vi "CheckForError.Test.vi"(0 "Main Path":path) -> (1 "Array of Folders":path[](array[path]), 2 "PRAMMS VRN":refnum<visa-resource-name>, 3 "Array of Files":path[](array[path]), 4 "SkipInstr":bool, 6 "Bundle-Meteo":T1={"cRIO address"="0.0.0.0", "Port Number"=0, "cRIO_commID"=refnum, "Cx"=FALSE}, 8 "This VI's Path":path, 10 "term":string, 11 "Go on ?":bool, 12 "Array of Baud Rates":u32[](array[numeric]), 13 "TCS-CommVRN":refnum<visa-resource-name>, 14 "Array of VISA refnum":refnum<visa-resource-name>[](array[refnum]), 15 "Serial":bool[](array[boolean]))   [LabVIEW 2011]
uses:
  Globals.vi
  <vilib>/Utility/config.llb/Read Key (U32).vi
  <vilib>/Utility/config.llb/Read Key (String).vi
  <vilib>/Instr/_visa.llb/VISA Configure Serial Port (Instr).vi
  Comm/SerialCommError.vi
  <vilib>/Utility/config.llb/Read Key (Path).vi
  <vilib>/Utility/config.llb/NI_LVConfig.lvlib
panel:
  in  "SkipInstr":bool
  out "Hexapode":bool
  out "Hexapod VRN":refnum<visa-resource-name>
  out "PRAMMS":bool
  out "ActiveDummy":bool
  out "TCS":bool
  out "TCP Error":errorcluster
  out "standard output":string
  out "standard error":string
  out "concatenated string":string
  out "Nettoyage":bool
  in  "restart":bool
  out "error out":errorcluster
  in  "cancel":bool
  in  "ignore":bool
  out "Master Dir":path
  out "IDL":bool
  out "wget":bool
  out "Ports Series":bool
  out "SubVIs":bool
  out "config error out":errorcluster
  out "Camera":bool
  out "Starry Night":bool
  out "Configuration":bool
  out "Arborescence":bool
  # "Version sans GUI de ErrorCheck.vi  Vérifie :\n    - Existence des chemins/fichiers nécessaire\n    - Communication avec les différents périphériques\n    - Lien ActiveX avec Starry Night\n    - Vérifie la communication avec la station météo\n    - Vérifie l'état de la face avant des VIs utilisés\n    - Compatibilité des versions installées\n    - Vérifie la disponibilité des applications (wget, IDL)"
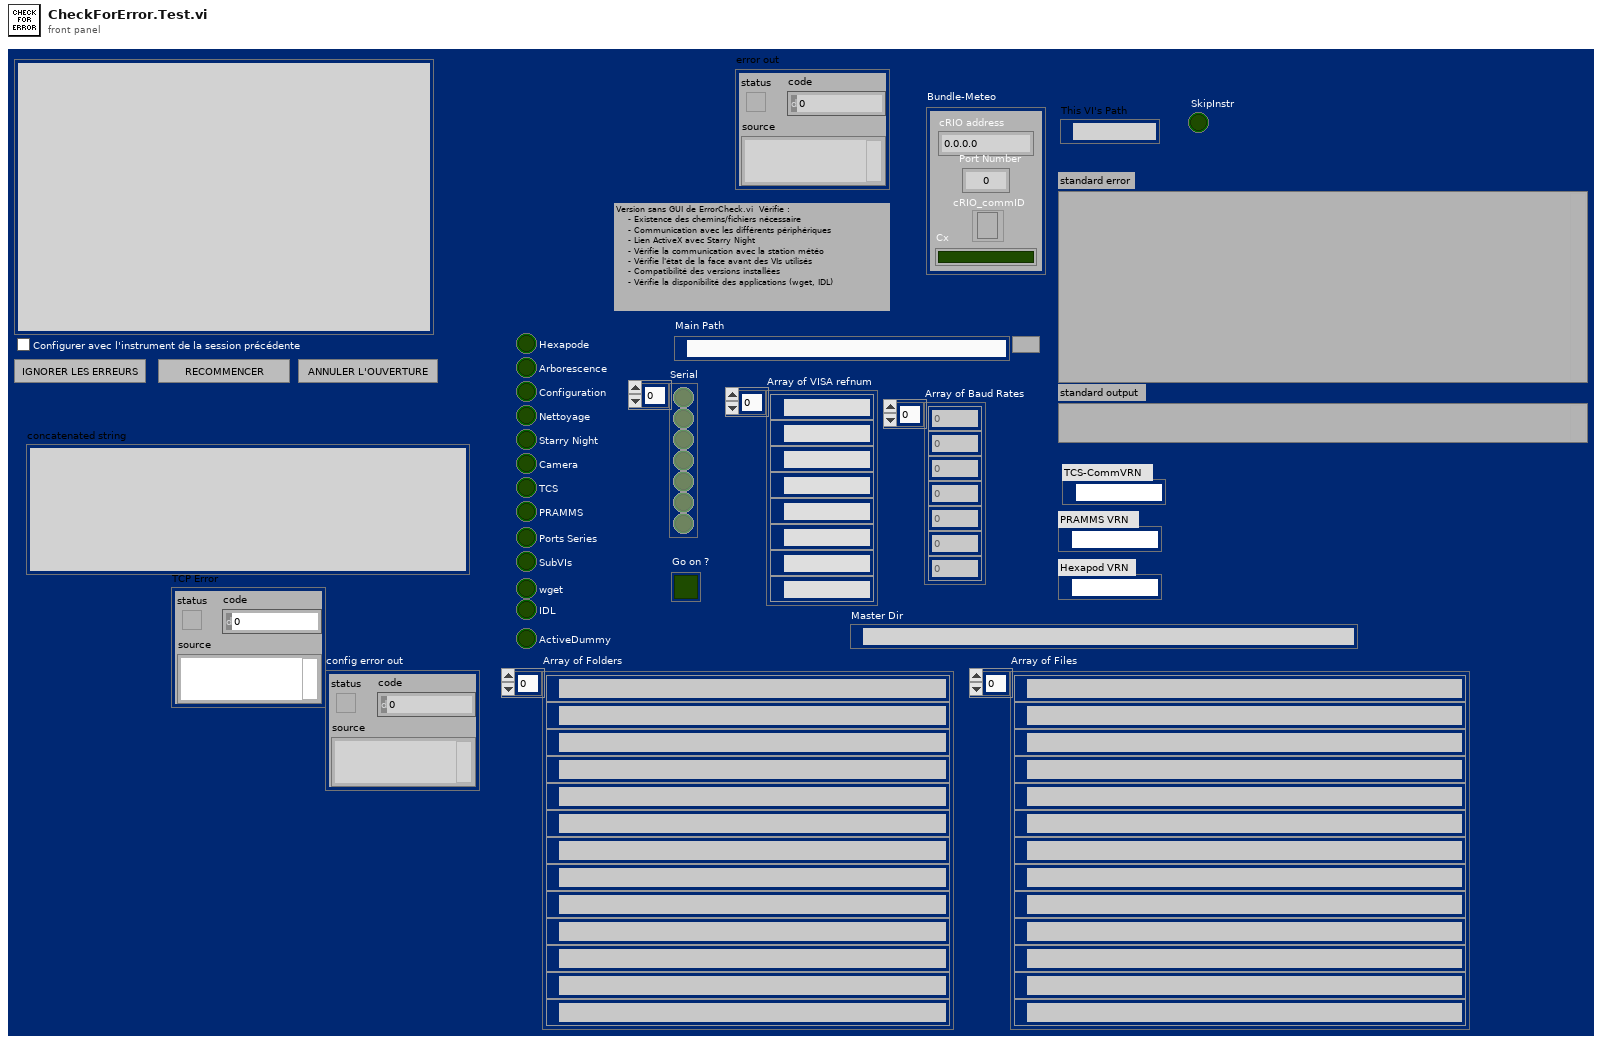
[diagram p1: front panel]
types:
  T1 = cluster{"cRIO address":string, "Port Number":u16, "cRIO_commID":refnum<k5>, "Cx":bool}
  T2 = enum8{"Enabled", "Disabled", "Disabled and Grayed Out"}
  T3 = typedef "NI_LVConfig.lvlib/Config Data RefNum.ctl" = refnum<k1>
  T4 = cluster{"value":string, u16, "connection ID":refnum<k5>, bool}
  T5 = enum16{"Left Button", "Center Button", "Right Button", "Window Close"}
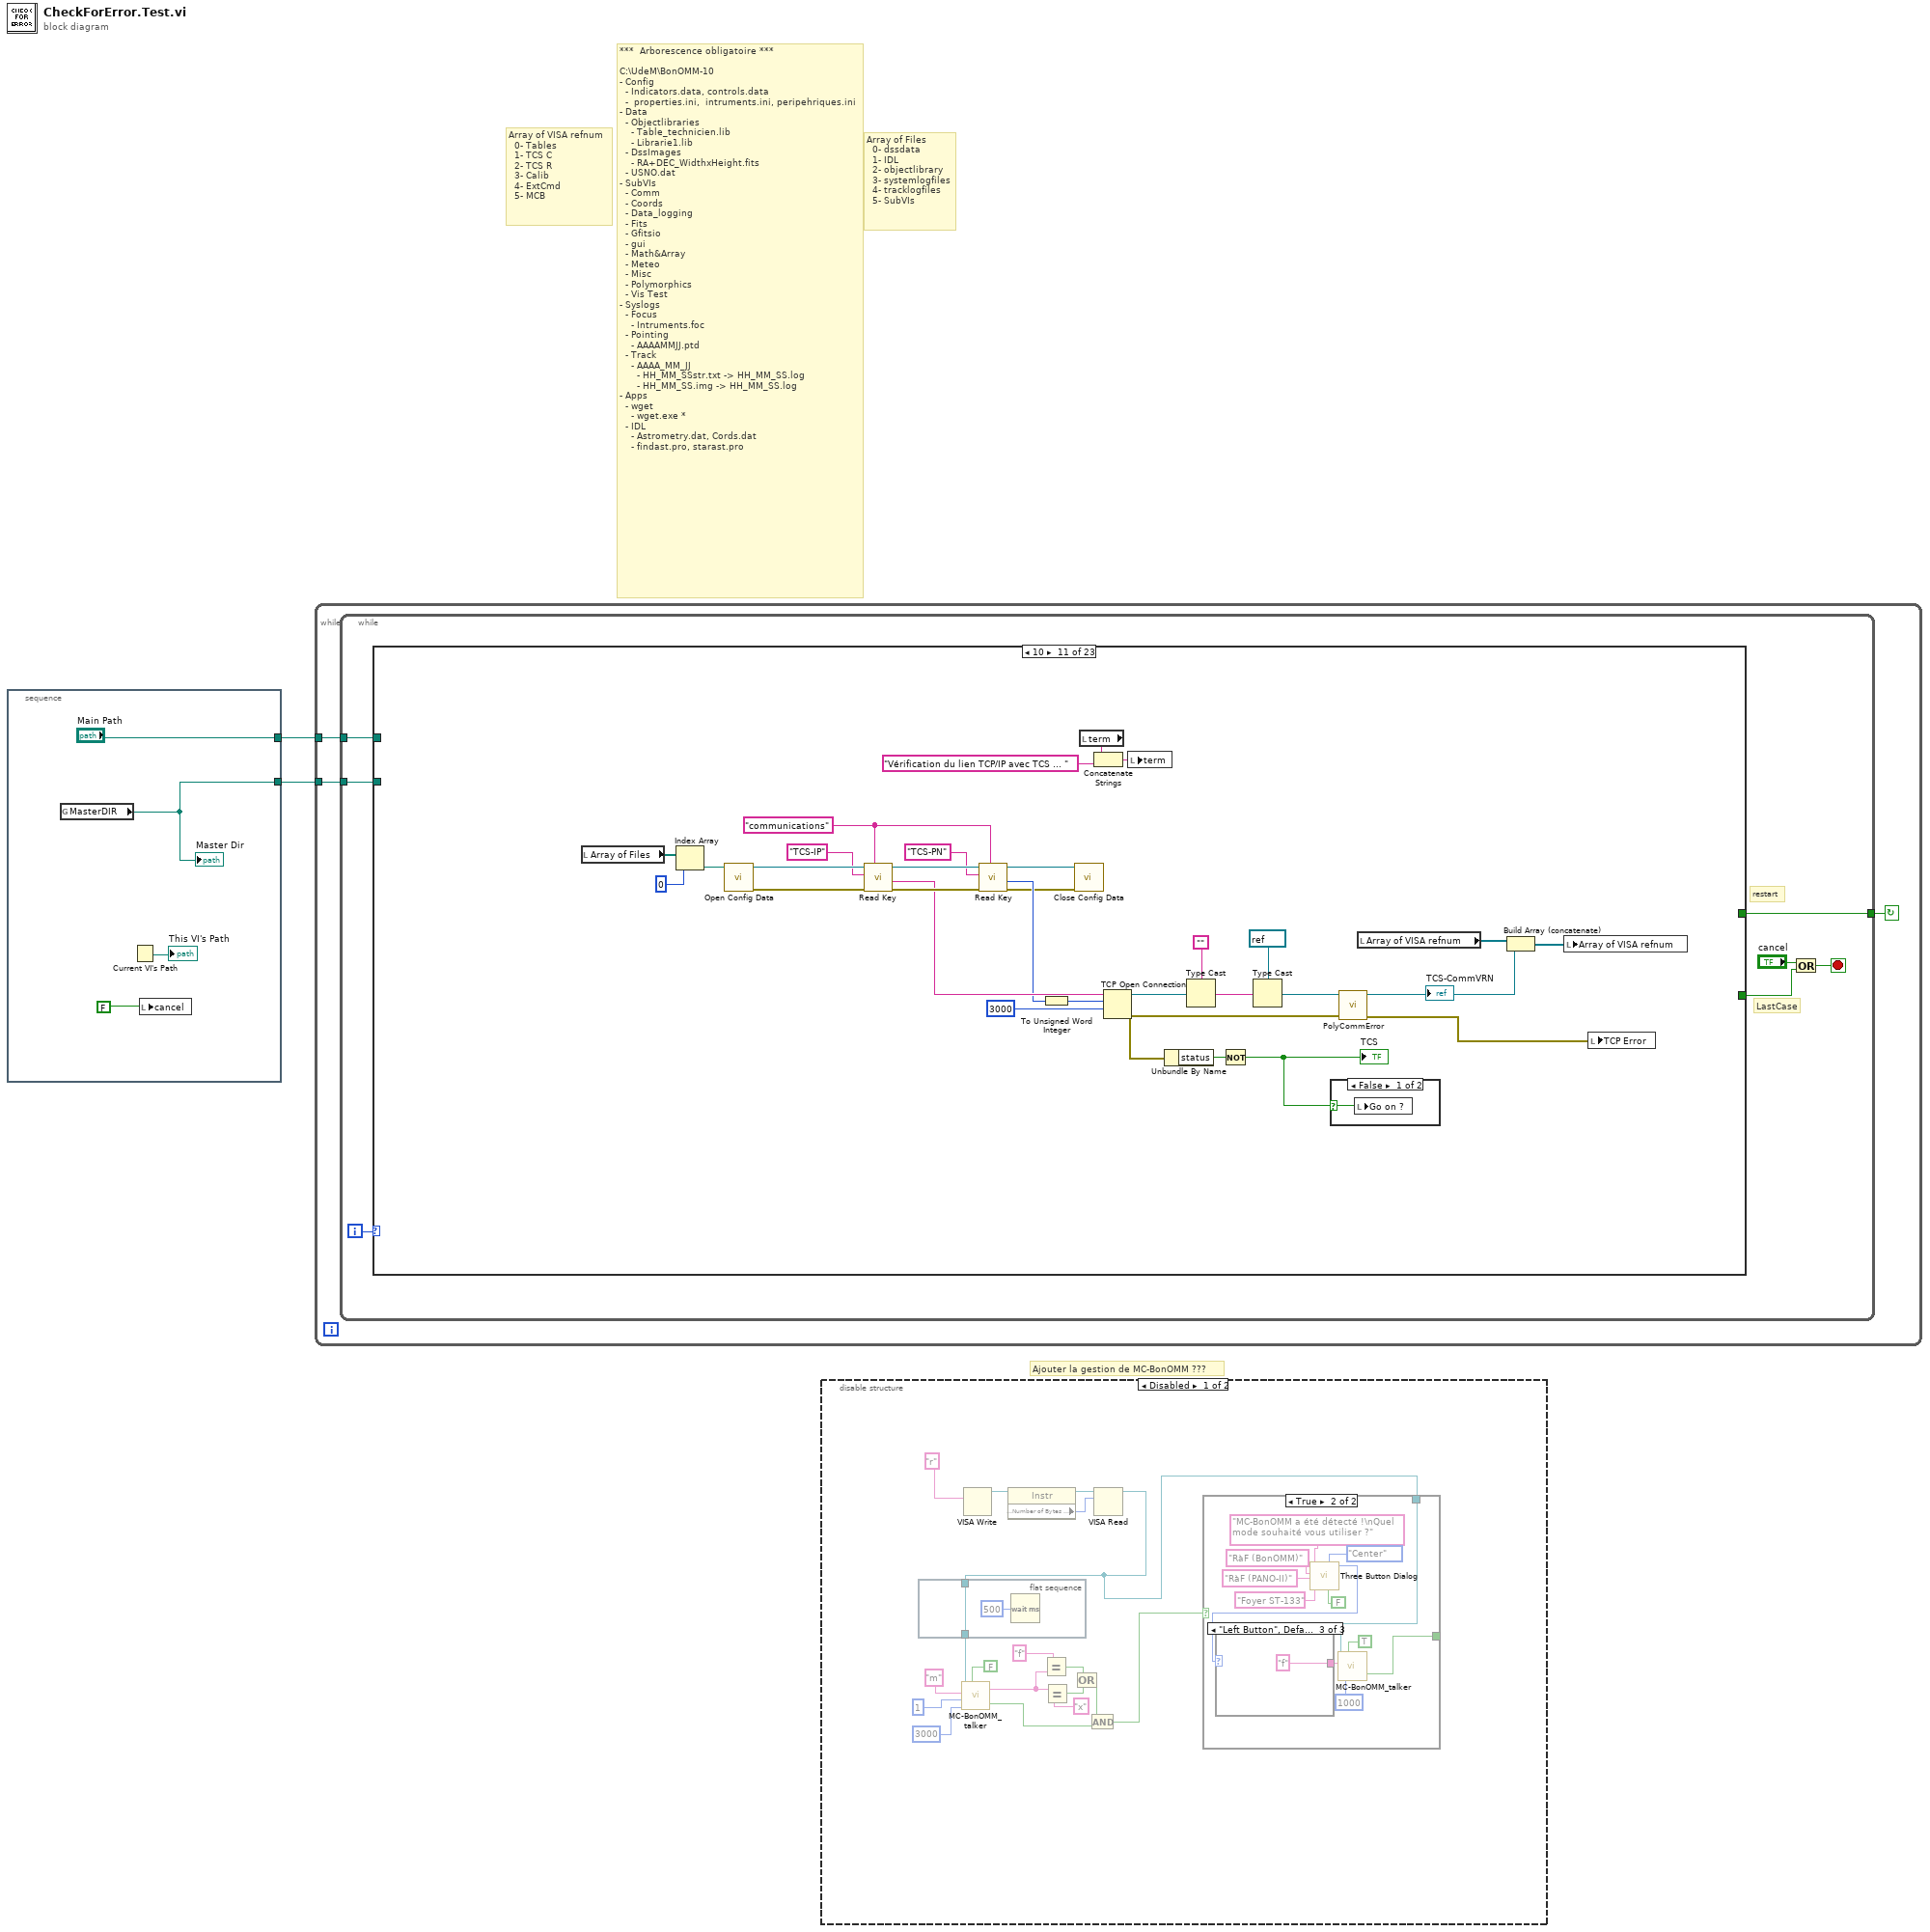
[diagram p0: block diagram]
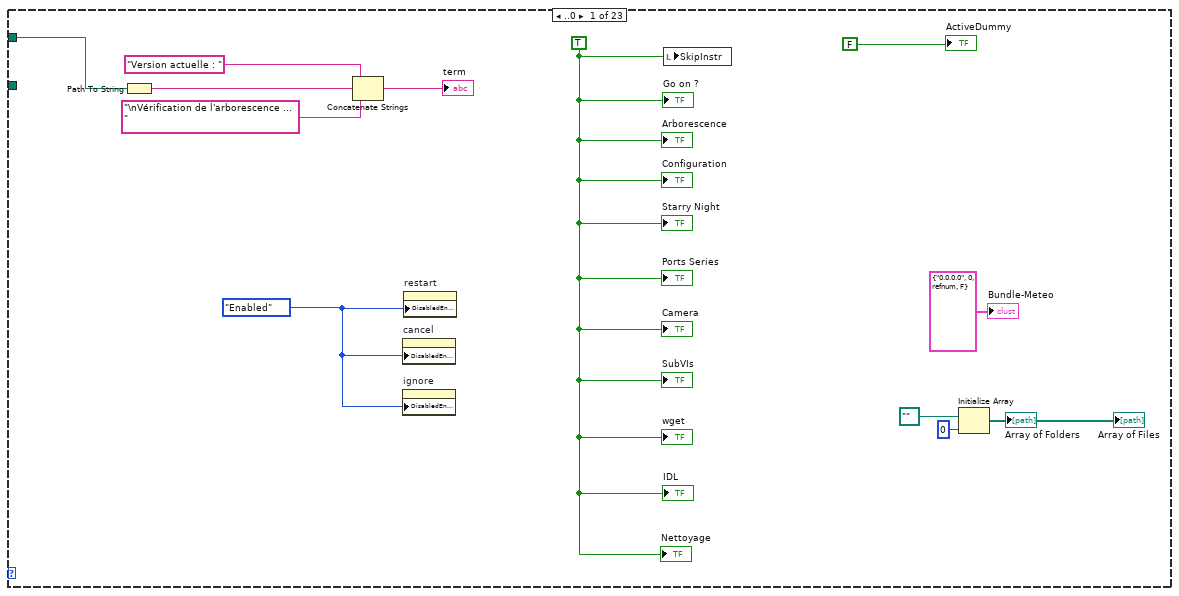
[diagram p2: hidden frame]
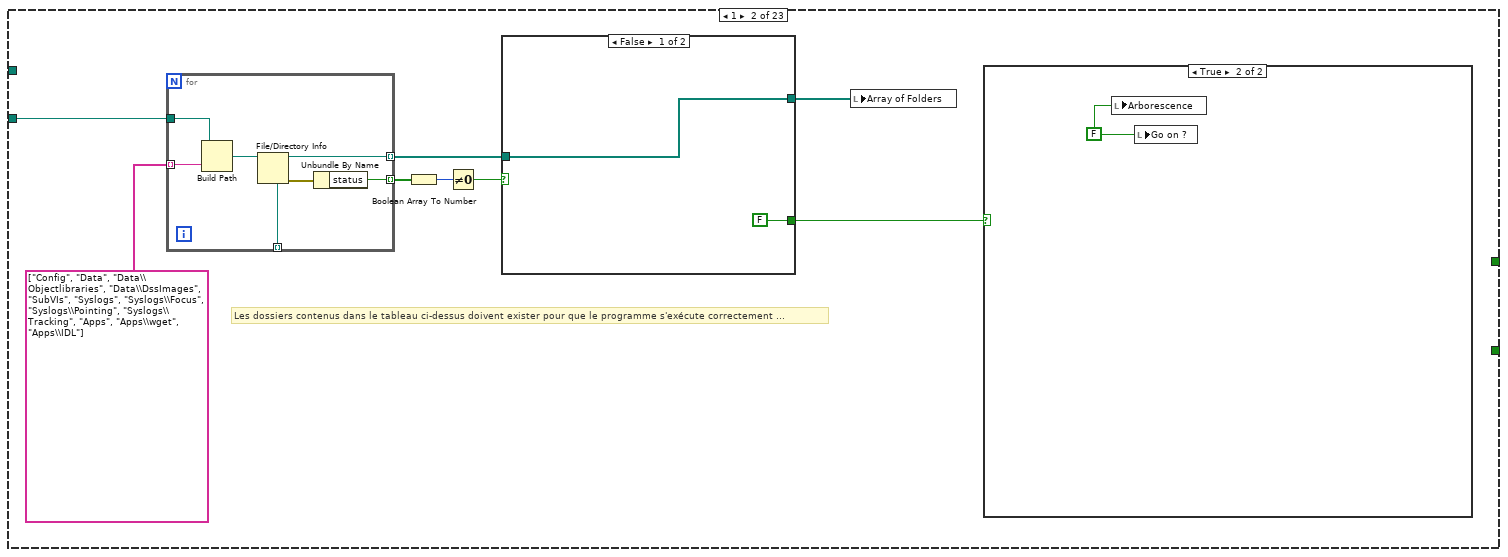
[diagram p3: hidden frame]
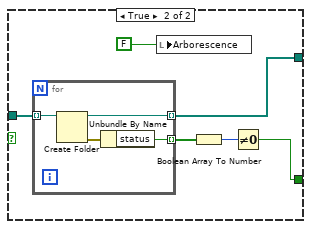
[diagram p5: hidden frame]
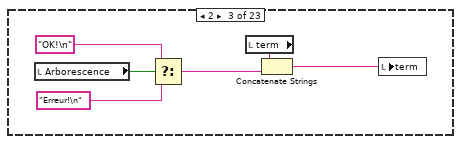
[diagram p6: hidden frame]
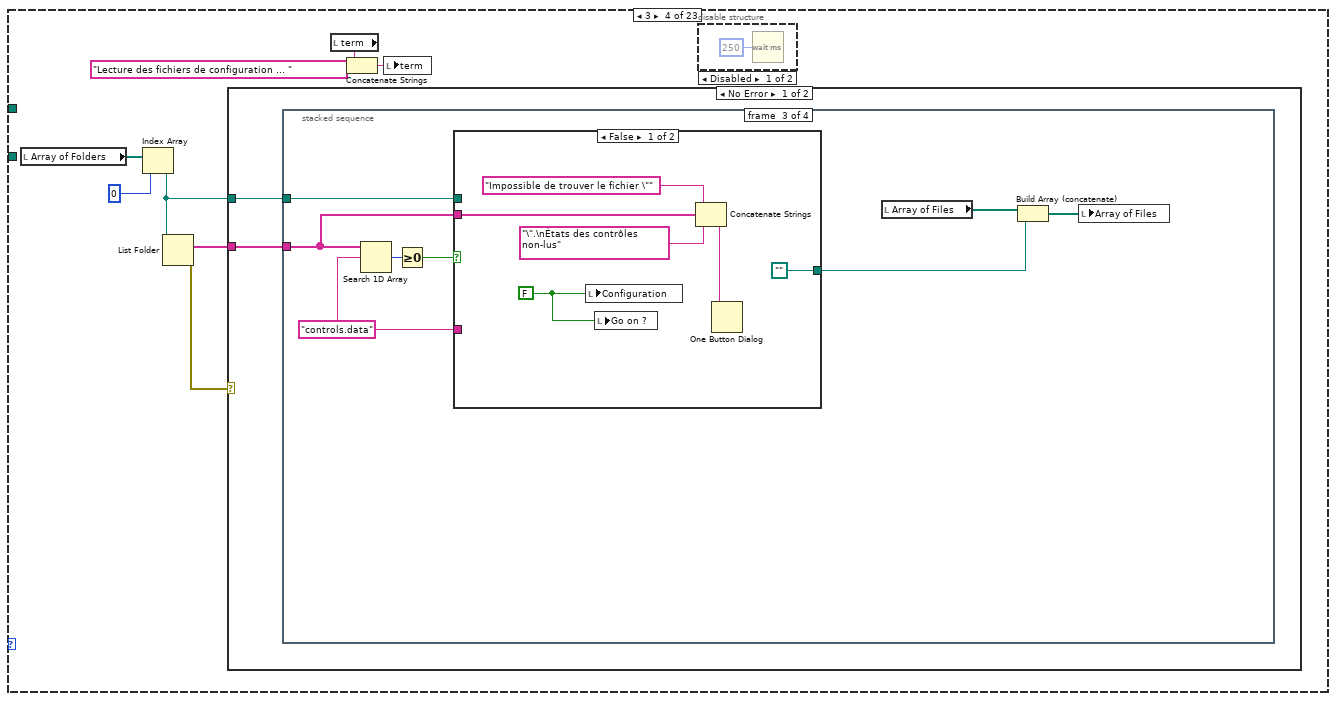
[diagram p7: hidden frame]
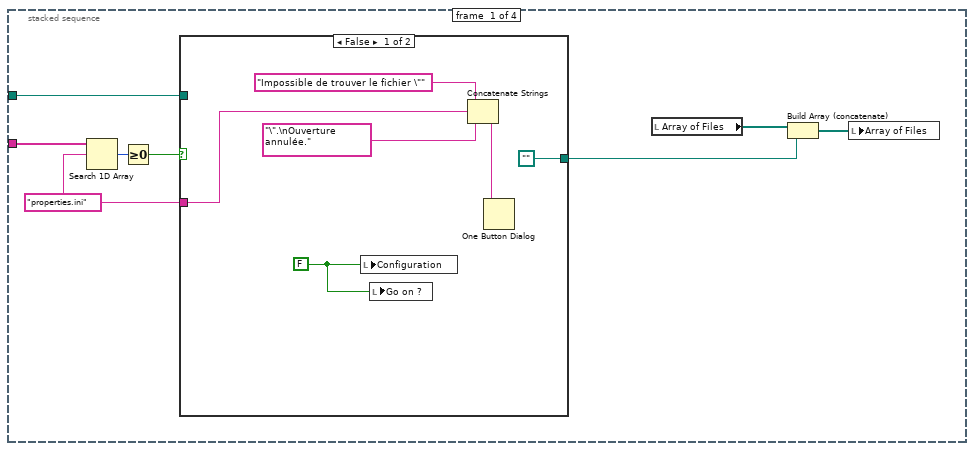
[diagram p9: hidden frame]
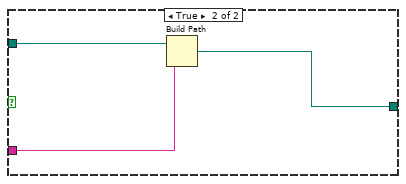
[diagram p10: hidden frame]
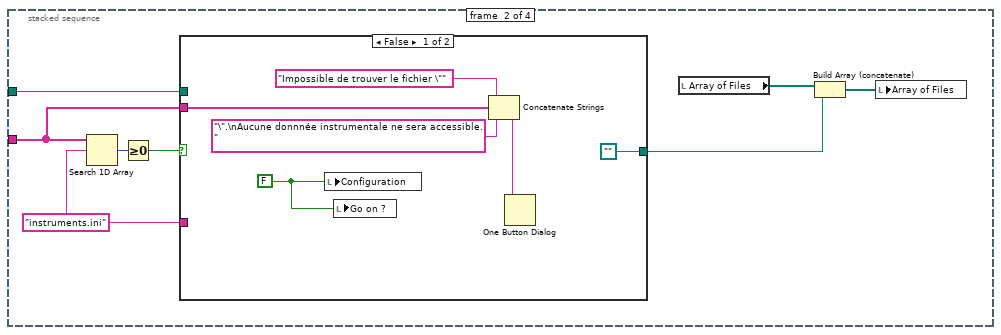
[diagram p11: hidden frame]
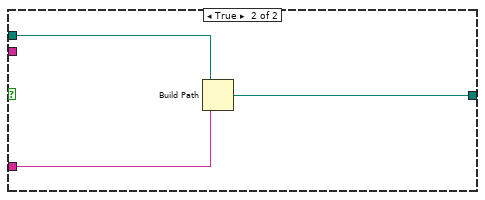
[diagram p12: hidden frame]
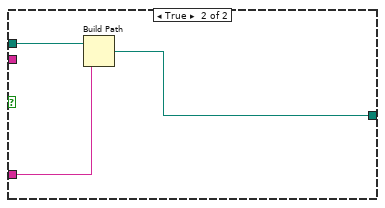
[diagram p13: hidden frame]
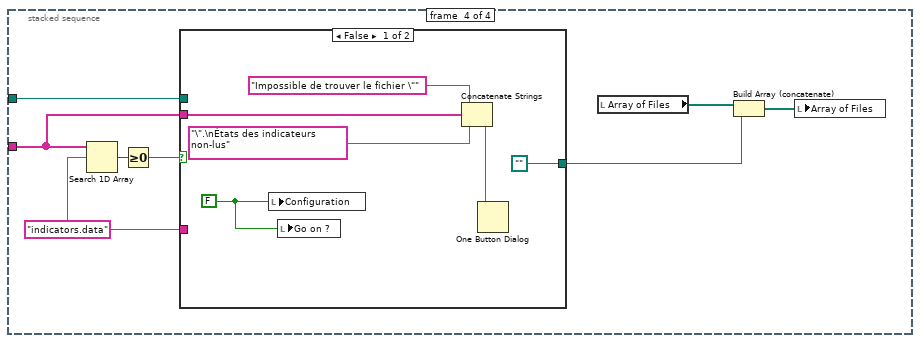
[diagram p14: hidden frame]
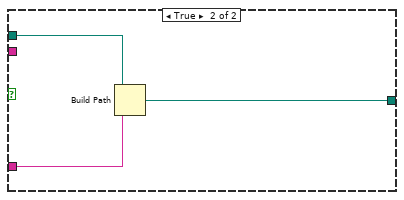
[diagram p15: hidden frame]
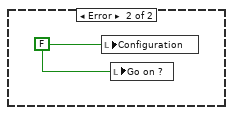
[diagram p16: hidden frame]
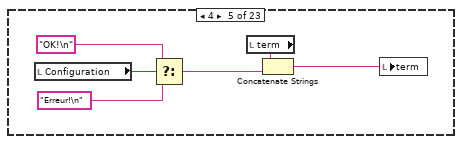
[diagram p17: hidden frame]
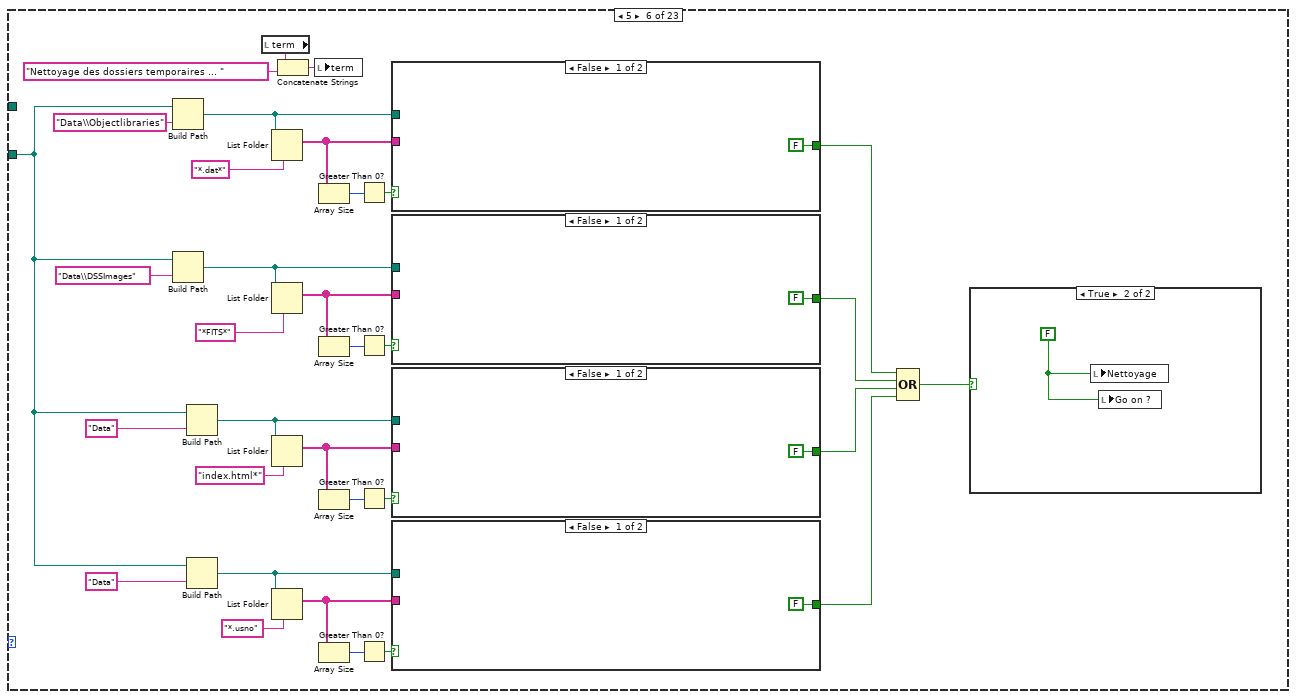
[diagram p18: hidden frame]
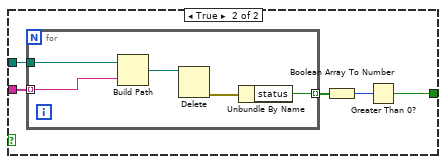
[diagram p19: hidden frame]
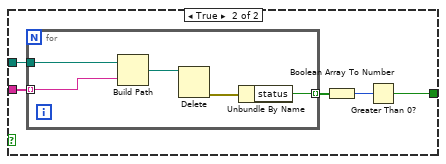
[diagram p20: hidden frame]
diagram:
  # "Array of Files\n  0- dssdata\n  1- IDL\n  2- objectlibrary\n  3- systemlogfiles\n  4- tracklogfiles\n  5- SubVIs"
  # "***  Arborescence obligatoire ***\n\nC:\\UdeM\\BonOMM-10\n-\tConfig\n  -\tIndicators.data, controls.data\n  -\t properties.ini,  intruments.ini, peripehriques.ini\n-\tData\n  -\tObjectlibraries\n    -\tTable_technicien.lib\n    -\tLibrarie1.lib\n  -\tDssImages\n    -\tRA+DEC_WidthxHeight.fits\n  -\tUSNO.dat\n-\tSubVIs\n  -\tComm\n  -\tCoords\n  -\tData_logging\n  -\tFits\n  -\tGfitsio\n  -\tgui\n  -\tMath&Array\n  -\tMeteo\n  -\tMisc\n  -\tPolymorphics\n  -\tVis Test\n-\tSyslogs\n  -\tFocus\n    -\tIntruments.foc\n  -\tPointing\n    -\tAAAAMMJJ.ptd\n  -\tTrack\n    -\tAAAA_MM_JJ\n      -\tHH_MM_SSstr.txt -> HH_MM_SS.log\n      -\tHH_MM_SS.img -> HH_MM_SS.log\n-\tApps\n  -\twget\n    -\twget.exe *\n  -\tIDL\n    -\tAstrometry.dat, Cords.dat\n    -\tfindast.pro, starast.pro"
  # "Array of VISA refnum\n  0- Tables\n  1- TCS C\n  2- TCS R\n  3- Calib\n  4- ExtCmd\n  5- MCB"
  # "Ajouter la gestion de MC-BonOMM ???"
  n1 = stacked-sequence {
    tunnel: ["Main Path"] -> w2
    tunnel: [w4] -> w1
    frame #0 {
      n2 = global read "Globals.vi" "MasterDIR"() -> (w4:path)
      "Master Dir" <- w4
      n3 = Current VI's Path() -> (path=→"This VI's Path":path)
      n4 = local write "cancel"(FALSE ("Arborescence")) -> ()
    }
  }
  n5 = while {
    tunnel: w2 -> [w9]
    tunnel: w1 -> [w8]
    stop <- w7 continue-if-true
    n6 = while {
      tunnel: w8 -> [w16]
      tunnel: w9 -> [w15]
      tunnel: [w11] -> w7
      i -> [w14]
      stop <- w12 stop-if-true
      # "LastCase"
      # "restart"
      n7 = case shown="10" w14 {
        tunnel: w16 -> [_ w35 _ _ _ w149 _ _ _ _ _ _ _ _ _ _ _ _ _ _ _ _ _]
        tunnel: w15 -> [w24 _ _ _ _ _ _ _ _ _ _ _ _ _ _ _ _ _ _ _ _ _ _]
        tunnel: [_ _ _ _ _ _ _ _ _ _ _ _ _ _ _ _ _ _ _ _ _ w687 _] -> w11
        tunnel: [_ _ _ _ _ _ _ _ _ _ _ _ _ _ _ _ _ _ _ _ _ w687 w714] -> w10
        frame ..0 {
          w19 = T2."Enabled" ("Disabled")
          w18 = TRUE ("Arborescence")
          n8 = Path To String(path=w24) -> (string=w28:string)
          n9 = Concatenate Strings("Version actuelle : ", w28, "\nVérification de l'arborescence ... ") -> (→"term":string)
          n10 = property on="cancel" class="Bool (strict)"("DisabledEnum"=w19) -> ()  [unwired: 2 in, 2 out]
          n11 = property on="ignore" class="Bool"("DisabledEnum"=w19) -> ()  [unwired: 2 in, 2 out]
          n12 = property on="restart" class="Bool"("DisabledEnum"=w19) -> ()  [unwired: 2 in, 2 out]
          n13 = local write "SkipInstr"(w18) -> ()
          n14 = Initialize Array(path "" ("path dup"), 0 ("dimension size")) -> (→"Array of Folders" →"Array of Files":path[])
          "Arborescence" <- w18
          "Configuration" <- w18
          "Starry Night" <- w18
          "Camera" <- w18
          "SubVIs" <- w18
          "Ports Series" <- w18
          "wget" <- w18
          "IDL" <- w18
          "Bundle-Meteo" <- T1 {"cRIO address"="0.0.0.0", "Port Number"=0, "cRIO_commID"=refnum, "Cx"=FALSE} ("Bundle-Meteo")
          "Nettoyage" <- w18
          "ActiveDummy" <- FALSE ("Arborescence")
          "Go on ?" <- w18
        }
        frame 1 {
          # "Les dossiers contenus dans le tableau ci-dessus doivent exister pour que le programme s'exécute correctement ..."
          n15 = for {
            tunnel: string[] ["Config", "Data", "Data\\Objectlibraries", "Data\\DssImages", "SubVIs", "Syslogs", "Syslogs\\Focus", "Syslogs\\Pointing", "Syslogs\\Tracking", "Apps", "Apps\\wget", "Apps\\IDL"] -> [w55] mode=indexing
            tunnel: w35 -> [w56]
            tunnel: [w53] -> w31 mode=indexing
            tunnel: [w52] -> _ mode=indexing
            tunnel: [w50] -> w34 mode=indexing
            n16 = Build Path(base path=w56, name or relative path=w55) -> (appended path=w54:path)
            n17 = File/Directory Info(path=w54) -> (path out=w53:path, error out=w51:errorcluster, resolved path=w52:path)  [unwired: 1 in, 4 out]
            n18 = Unbundle By Name(w51) -> ("status"=w50:bool)
          }
          n19 = Boolean Array To Number(Boolean array=w34) -> (number=w33:u32)
          n20 = Not Equal To 0?(x=w33) -> (x != 0?=w32:bool)
          n21 = case shown="False" w32 {
            tunnel: w31 -> [w38 w45]
            tunnel: [FALSE w42] -> w30
            tunnel: [w38 w41] -> w29
            frame False {
            }
            frame True {
              n22 = for {
                tunnel: w45 -> [w49] mode=indexing
                tunnel: [w47] -> w43 mode=indexing
                tunnel: [w46] -> w41 mode=indexing
                n23 = Create Folder(path (use dialog)=w49) -> (created path=w46:path, error out=w48:errorcluster)  [unwired: 2 in, 1 out]
                n24 = Unbundle By Name(w48) -> ("status"=w47:bool)
              }
              n25 = local write "Arborescence"(FALSE) -> ()
              n26 = Boolean Array To Number(Boolean array=w43) -> (number=w44:u32)
              n27 = Not Equal To 0?(x=w44) -> (x != 0?=w42:bool)
            }
          }
          n28 = local write "Array of Folders"(w29) -> ()
          n29 = case shown="True" w30 {
            frame False {
            }
            frame True {
              w37 = FALSE
              n30 = local write "Arborescence"(w37) -> ()
              n31 = local write "Go on ?"(w37) -> ()
            }
          }
        }
        frame 2 {
          n32 = local read "Arborescence"() -> (w59:bool)
          n33 = Select(t="OK!\n" ("string"), s=w59, f="Erreur!\n" ("string")) -> (s? t:f=w60:string)
          n34 = local read "term"() -> (w61:string)
          n35 = Concatenate Strings(w61, w60) -> (w62:string)
          n36 = local write "term"(w62) -> ()
        }
        frame 3 {
          n37 = local read "Array of Folders"() -> (w65:path[])
          n38 = Index Array(array=w65, index=0) -> (element=w63:path)
          n39 = List Folder(path=w63) -> (filenames=w67:string[], error out=w66:errorcluster)  [unwired: 3 in, 2 out]
          n40 = case shown="No Error" w66 {
            tunnel: w67 -> [w73 _]
            tunnel: w63 -> [w72 _]
            frame No Error {
              n41 = stacked-sequence {
                tunnel: w73 -> [w79 w96 w113 w130]
                tunnel: w72 -> [w76 w94 w112 w129]
                frame #0 {
                  w75 = "properties.ini"
                  n42 = Search 1D Array(1D array=w79, element=w75) -> (index of element=w81:i32)  [unwired: 1 in]
                  n43 = Greater Or Equal To 0?(x=w81) -> (x >= 0?=w80:bool)
                  n44 = case shown="False" w80 {
                    tunnel: w76 -> [_ w90]
                    tunnel: w75 -> [w83 w89]
                    tunnel: [path "" w88] -> w74
                    frame False {
                      w84 = FALSE ("Configuration")
                      n45 = local write "Configuration"(w84) -> ()
                      n46 = local write "Go on ?"(w84) -> ()
                      n47 = Concatenate Strings("Impossible de trouver le fichier \"", w83, "\".\nOuverture annulée.") -> (w85:string)
                      n48 = One Button Dialog(message=w85) -> ()  [unwired: 1 in, 1 out]
                    }
                    frame True {
                      n49 = Build Path(base path=w90, name or relative path=w89) -> (appended path=w88:path)
                    }
                  }
                  n50 = local read "Array of Files"() -> (w78:path[])
                  n51 = Build Array (concatenate)(w78, w74) -> (w77:path[])
                  n52 = local write "Array of Files"(w77) -> ()
                }
                frame #1 {
                  w95 = "instruments.ini"
                  n53 = Search 1D Array(1D array=w96, element=w95) -> (index of element=w98:i32)  [unwired: 1 in]
                  n54 = Greater Or Equal To 0?(x=w98) -> (x >= 0?=w97:bool)
                  n55 = case shown="False" w97 {
                    tunnel: w96 -> [w102 _]
                    tunnel: w95 -> [_ w107]
                    tunnel: w94 -> [_ w106]
                    tunnel: [path "" w105] -> w91
                    frame False {
                      w100 = FALSE ("Configuration")
                      n56 = local write "Configuration"(w100) -> ()
                      n57 = local write "Go on ?"(w100) -> ()
                      n58 = Concatenate Strings("Impossible de trouver le fichier \"", w102, "\".\nAucune donnnée instrumentale ne sera accessible.") -> (w101:string)
                      n59 = One Button Dialog(message=w101) -> ()  [unwired: 1 in, 1 out]
                    }
                    frame True {
                      n60 = Build Path(base path=w106, name or relative path=w107) -> (appended path=w105:path)
                    }
                  }
                  n61 = local read "Array of Files"() -> (w93:path[])
                  n62 = Build Array (concatenate)(w93, w91) -> (w92:path[])
                  n63 = local write "Array of Files"(w92) -> ()
                }
                frame #2 {
                  w111 = "controls.data"
                  n64 = Search 1D Array(1D array=w113, element=w111) -> (index of element=w115:i32)  [unwired: 1 in]
                  n65 = Greater Or Equal To 0?(x=w115) -> (x >= 0?=w114:bool)
                  n66 = case shown="False" w114 {
                    tunnel: w113 -> [w119 _]
                    tunnel: w112 -> [_ w124]
                    tunnel: w111 -> [_ w123]
                    tunnel: [path "" w122] -> w108
                    frame False {
                      w117 = FALSE ("Configuration")
                      n67 = local write "Configuration"(w117) -> ()
                      n68 = local write "Go on ?"(w117) -> ()
                      n69 = Concatenate Strings("Impossible de trouver le fichier \"", w119, "\".\nÉtats des contrôles non-lus") -> (w118:string)
                      n70 = One Button Dialog(message=w118) -> ()  [unwired: 1 in, 1 out]
                    }
                    frame True {
                      n71 = Build Path(base path=w124, name or relative path=w123) -> (appended path=w122:path)
                    }
                  }
                  n72 = local read "Array of Files"() -> (w110:path[])
                  n73 = Build Array (concatenate)(w110, w108) -> (w109:path[])
                  n74 = local write "Array of Files"(w109) -> ()
                }
                frame #3 {
                  w128 = "indicators.data"
                  n75 = Search 1D Array(1D array=w130, element=w128) -> (index of element=w132:i32)  [unwired: 1 in]
                  n76 = Greater Or Equal To 0?(x=w132) -> (x >= 0?=w131:bool)
                  n77 = case shown="False" w131 {
                    tunnel: w130 -> [w136 _]
                    tunnel: w129 -> [_ w141]
                    tunnel: w128 -> [_ w140]
                    tunnel: [path "" w139] -> w125
                    frame False {
                      w134 = FALSE ("Configuration")
                      n78 = local write "Configuration"(w134) -> ()
                      n79 = local write "Go on ?"(w134) -> ()
                      n80 = Concatenate Strings("Impossible de trouver le fichier \"", w136, "\".\nÉtats des indicateurs non-lus") -> (w135:string)
                      n81 = One Button Dialog(message=w135) -> ()  [unwired: 1 in, 1 out]
                    }
                    frame True {
                      n82 = Build Path(base path=w141, name or relative path=w140) -> (appended path=w139:path)
                    }
                  }
                  n83 = local read "Array of Files"() -> (w127:path[])
                  n84 = Build Array (concatenate)(w127, w125) -> (w126:path[])
                  n85 = local write "Array of Files"(w126) -> ()
                }
              }
            }
            frame Error {
              w142 = FALSE ("Configuration")
              n86 = local write "Configuration"(w142) -> ()
              n87 = local write "Go on ?"(w142) -> ()
            }
          }
          n88 = local read "term"() -> (w69:string)
          n89 = Concatenate Strings(w69, "Lecture des fichiers de configuration ... " ("string")) -> (w70:string)
          n90 = local write "term"(w70) -> ()
          n91 = disable-structure shown="Disabled" {
            frame Disabled {
              n92 = Wait (ms)(milliseconds to wait=u32 250) -> ()  [unwired: 1 out]
            }
            frame Enabled {
            }
          }
        }
        frame 4 {
          n93 = local read "Configuration"() -> (w145:bool)
          n94 = Select(t="OK!\n" ("string"), s=w145, f="Erreur!\n" ("string")) -> (s? t:f=w146:string)
          n95 = local read "term"() -> (w147:string)
          n96 = Concatenate Strings(w147, w146) -> (w148:string)
          n97 = local write "term"(w148) -> ()
        }
        frame 5 {
          n98 = Build Path(base path=w149, name or relative path="Data\\Objectlibraries") -> (appended path=w174:path)
          n99 = Build Path(base path=w149, name or relative path="Data\\DSSImages") -> (appended path=w172:path)
          n100 = Build Path(base path=w149, name or relative path="Data") -> (appended path=w158:path)
          n101 = Build Path(base path=w149, name or relative path="Data") -> (appended path=w155:path)
          n102 = local read "term"() -> (w180:string)
          n103 = List Folder(path=w174, pattern="*.dat*") -> (filenames=w176:string[])  [unwired: 2 in, 3 out]
          n104 = List Folder(path=w172, pattern="*FITS*") -> (filenames=w170:string[])  [unwired: 2 in, 3 out]
          n105 = List Folder(path=w158, pattern="index.html*") -> (filenames=w160:string[])  [unwired: 2 in, 3 out]
          n106 = List Folder(path=w155, pattern="*.usno") -> (filenames=w154:string[])  [unwired: 2 in, 3 out]
          n107 = Concatenate Strings(w180, "Nettoyage des dossiers temporaires ... " ("string")) -> (w181:string)
          n108 = local write "term"(w181) -> ()
          n109 = Array Size(array=w176) -> (size(s)=w177:i32)
          n110 = Array Size(array=w170) -> (size(s)=w169:i32)
          n111 = Array Size(array=w160) -> (size(s)=w161:i32)
          n112 = Array Size(array=w154) -> (size(s)=w153:i32)
          n113 = Greater Than 0?(x=w177) -> (x > 0?=w178:bool)
          n114 = Greater Than 0?(x=w169) -> (x > 0?=w168:bool)
          n115 = Greater Than 0?(x=w161) -> (x > 0?=w162:bool)
          n116 = Greater Than 0?(x=w153) -> (x > 0?=w152:bool)
          n117 = case shown="False" w178 {
            tunnel: w176 -> [_ w220]
            tunnel: w174 -> [_ w219]
            tunnel: [FALSE w216] -> w166
            frame False {
            }
            frame True {
              n118 = for {
                tunnel: w220 -> [w224] mode=indexing
                tunnel: w219 -> [w225]
                tunnel: [w221] -> w218 mode=indexing
                n119 = Build Path(base path=w225, name or relative path=w224) -> (appended path=w223:path)
                n120 = Delete(path (use dialog)=w223) -> (error out=w222:errorcluster)  [unwired: 4 in, 2 out]
                n121 = Unbundle By Name(w222) -> ("status"=w221:bool)
              }
              n122 = Boolean Array To Number(Boolean array=w218) -> (number=w217:u32)
              n123 = Greater Than 0?(x=w217) -> (x > 0?=w216:bool)
            }
          }
          n124 = case shown="False" w168 {
            tunnel: w170 -> [_ w209]
            tunnel: w172 -> [_ w208]
            tunnel: [FALSE w205] -> w165
            frame False {
            }
            frame True {
              n125 = for {
                tunnel: w209 -> [w213] mode=indexing
                tunnel: w208 -> [w214]
                tunnel: [w210] -> w207 mode=indexing
                n126 = Build Path(base path=w214, name or relative path=w213) -> (appended path=w212:path)
                n127 = Delete(path (use dialog)=w212) -> (error out=w211:errorcluster)  [unwired: 4 in, 2 out]
                n128 = Unbundle By Name(w211) -> ("status"=w210:bool)
              }
              n129 = Boolean Array To Number(Boolean array=w207) -> (number=w206:u32)
              n130 = Greater Than 0?(x=w206) -> (x > 0?=w205:bool)
            }
          }
          n131 = case shown="False" w162 {
            tunnel: w160 -> [_ w198]
            tunnel: w158 -> [_ w197]
            tunnel: [FALSE w194] -> w159
            frame False {
            }
            frame True {
              n132 = for {
                tunnel: w198 -> [w202] mode=indexing
                tunnel: w197 -> [w203]
                tunnel: [w199] -> w196 mode=indexing
                n133 = Build Path(base path=w203, name or relative path=w202) -> (appended path=w201:path)
                n134 = Delete(path (use dialog)=w201) -> (error out=w200:errorcluster)  [unwired: 4 in, 2 out]
                n135 = Unbundle By Name(w200) -> ("status"=w199:bool)
              }
              n136 = Boolean Array To Number(Boolean array=w196) -> (number=w195:u32)
              n137 = Greater Than 0?(x=w195) -> (x > 0?=w194:bool)
            }
          }
          n138 = case shown="False" w152 {
            tunnel: w154 -> [_ w187]
            tunnel: w155 -> [_ w186]
            tunnel: [FALSE w183] -> w150
            frame False {
            }
            frame True {
              n139 = for {
                tunnel: w187 -> [w191] mode=indexing
                tunnel: w186 -> [w192]
                tunnel: [w188] -> w185 mode=indexing
                n140 = Build Path(base path=w192, name or relative path=w191) -> (appended path=w190:path)
                n141 = Delete(path (use dialog)=w190) -> (error out=w189:errorcluster)  [unwired: 4 in, 2 out]
                n142 = Unbundle By Name(w189) -> ("status"=w188:bool)
              }
              n143 = Boolean Array To Number(Boolean array=w185) -> (number=w184:u32)
              n144 = Greater Than 0?(x=w184) -> (x > 0?=w183:bool)
            }
          }
          n145 = Compound Arithmetic op=OR(w166, w165, w159, w150) -> (w167:bool)
          n146 = case shown="True" w167 {
            frame False {
            }
            frame True {
              w226 = FALSE
              n147 = local write "Nettoyage"(w226) -> ()
              n148 = local write "Go on ?"(w226) -> ()
            }
          }
        }
        frame 6 {
          n149 = local read "Nettoyage"() -> (w229:bool)
          n150 = Select(t="OK!\n" ("string"), s=w229, f="Erreur!\n" ("string")) -> (s? t:f=w230:string)
          n151 = local read "term"() -> (w231:string)
          n152 = Concatenate Strings(w231, w230) -> (w232:string)
          n153 = local write "term"(w232) -> ()
        }
        frame 7 {
          n154 = local read "term"() -> (w239:string)
          n155 = Concatenate Strings(w239, "Test du lien ActiveX avec Starry Night ... " ("string")) -> (w240:string)
          n156 = local write "term"(w240) -> ()
          n157 = Automation Open(Automation Refnum=refnum<k7> refnum ("ScopeSim._Telescope")) -> (Automation Refnum=w233:refnum<k7>, error out=w236:errorcluster)  [unwired: 3 in]
          n158 = Unbundle By Name(w236) -> ("status"=w235:bool)
          n159 = case shown="True" w235 {
            tunnel: w233 -> [w243 _]
            tunnel: [w242 FALSE ("Connected")] -> w237
            frame False {
              n160 = property class="_Telescope"(reference=w243) -> (reference out=w241:refnum<k7>, "Connected"=w242:bool)  [unwired: 1 in, 1 out]
              n161 = Close Reference(reference=w241) -> ()  [unwired: 1 in, 1 out]
            }
            frame True {
            }
          }
          n162 = global write "Globals.vi" "ScopeSim._Telescope"(w233) -> ()
          n163 = case shown="True" w237 {
            frame False {
              w245 = FALSE
              n164 = local write "Starry Night"(w245) -> ()
              n165 = local write "Go on ?"(w245) -> ()
            }
            frame True {
            }
          }
        }
        frame 8 {
          n166 = local read "Starry Night"() -> (w246:bool)
          n167 = Select(t="OK!\n" ("string"), s=w246, f="Erreur!\n" ("string")) -> (s? t:f=w249:string)
          n168 = local read "term"() -> (w250:string)
          n169 = Concatenate Strings(w250, w249) -> (w251:string)
          n170 = local write "term"(w251) -> ()
        }
        frame 9 {
          n171 = local read "Array of Files"() -> (w254:path[])
          n172 = Index Array(array=w254, index=0) -> (element=w253:path)
          n173 = call <vilib>:"Open Config Data.vi"("configuration file path"=w253) -> ("error out"=w262:errorcluster, "refnum"=w264:T3)  [unwired: 8 in, 1 out]
          n174 = for {
            tunnel: string[] ["tablespd", "calibspd", "excspd", "mcbspd", "splspd"] -> [w285] mode=indexing
            tunnel: string[] ["tablevrn", "calibvrn", "excvrn", "mcbvrn", "splvrn"] -> [w284] mode=indexing
            tunnel: "communications" -> [w277]
            tunnel: w264 -> [w287]
            tunnel: [w286] -> w263
            shift-right: [w282] -> w261
            shift-left: w262 -> [w283]
            tunnel: [w274] -> w257 mode=indexing
            tunnel: [w276] -> w256 mode=indexing
            tunnel: [w270] -> w255 mode=indexing
            tunnel: [w272] -> _ mode=indexing
            i -> [w278]
            n175 = call-poly <vilib>:"Read Key.vi"("section"=w277, "error in (no error)"=w283, "default value"=u32 9600, "key"=w285, "refnum"=w287) -> ("error out"=w288:errorcluster, "value"=w270:u32, "refnum out"=w289:T3)  [unwired: 3 in, 1 out]
            n176 = call-poly <vilib>:"Read Key.vi"("section"=w277, "error in (no error)"=w288, "default value"="-1", "key"=w284, "refnum"=w289) -> ("error out"=w282:errorcluster, "value"=w273:string, "refnum out"=w286:T3)  [unwired: 3 in, 1 out]
            n177 = Type Cast(type=refnum<visa-resource-name> "-1" ("Table VRN"), x=w273) -> (*(type *) &x=w271:refnum<visa-resource-name>)
            n178 = case shown="0" w278 {
              tunnel: w271 -> [_ w318 w327 w348 w364 w385]
              tunnel: [refnum<visa-resource-name> "-1" ("Table VRN") w310 w339 w346 w362 w382] -> w275
              tunnel: [FALSE ("ok ?") w314 w340 w358 w369 w384] -> w276
              tunnel: w273 -> [_ w322 w334 w353 w370 w381]
              tunnel: w270 -> [_ w312 w329 w347 w363 w376]
              tunnel: [errorcluster {"status"=FALSE, "code"=0, "source"=""} ("error out") w307 w326 w345 w361 w383] -> w269
              frame -1, Default {
                (unwired) "Bizzarerie ... " ("string")
              }
              frame 0 {
                n179 = control-ref of="ActiveDummy"() -> (w306:refnum<vi>)
                n180 = Equal?(x=refnum<visa-resource-name> "N/A" ("Table VRN"), y=w318) -> (x = y?=w316:bool)
                n181 = Select(t=refnum<visa-resource-name> "-1", s=w316, f=w318) -> (s? t:f=w313:refnum<visa-resource-name>)
                n182 = call "Newmark-Initialize.vi"("VISA resource name"=w313, "ActiveStages"=string[] ["AX", "AY", "AZ"], "baud rate"=w312, "Timeout"=u32 1000, "Bool Refnum"=w306) -> ("VISA resource name out"=w310:refnum<visa-resource-name>, "Error?"=w309:bool, "Error OUT"=w307:errorcluster)  [unwired: 8 in]
                n183 = Not(x=w316) -> (.not. x?=w317:bool)
                n184 = local read "term"() -> (w325:string)
                n185 = Concatenate Strings(w325, "   Table de guidage (" ("string"), w322, ") ... " ("string")) -> (w324:string)
                n186 = And(x=w309, y=w317) -> (x .and. y?=w315:bool)
                n187 = Not(x=w315) -> (.not. x?=w314:bool)
                n188 = local write "term"(w324) -> ()
              }
              frame 1 {
                w333 = u16 0 items=["None", "XON/XOFF", "RTS/CTS", "XON/XOFF & RTS/CTS", "DTR/DSR", "XON/XOFF & DTR/DSR"] ("flow control (0:none)")
                w332 = u16 10 items=["1.0"=10, "1.5"=15, "2.0"=20] ("stop bits (10: 1 bit)")
                n189 = call-poly "VISA Configure Serial Port"("VISA resource name"=w327, "baud rate (9600)"=w329, "data bits (8)"=u16 8, "parity (0:none)"=enum16{"None", "Odd", "Even", "Mark", "Space"}."None", "stop bits (10: 1 bit)"=w332, "flow control (0:none)"=w333) -> ("VISA resource name out"=w328:refnum<visa-resource-name>, "error out"=w326:errorcluster)  [unwired: 8 in]
                n190 = call "Controle_des_lampe.vi"("VISA resource name"=w328, "Status In"=bool[] [FALSE, FALSE, FALSE]) -> ("VISA resource name dup"=w339:refnum<visa-resource-name>, "Status Out"=w343:bool[])  [unwired: 1 out]
                n191 = local read "term"() -> (w338:string)
                n192 = Concatenate Strings(w338, "   Module de caibration (" ("string"), w334, ") ... " ("string")) -> (w337:string)
                n193 = Boolean Array To Number(Boolean array=w343) -> (number=w341:u32)
                n194 = Equal To 0?(x=w341) -> (x = 0?=w340:bool)
                n195 = local write "term"(w337) -> ()
              }
              frame 2 {
                w352 = u16 0 items=["None", "XON/XOFF", "RTS/CTS", "XON/XOFF & RTS/CTS", "DTR/DSR", "XON/XOFF & DTR/DSR"] ("flow control (0:none)")
                w351 = u16 10 items=["1.0"=10, "1.5"=15, "2.0"=20] ("stop bits (10: 1 bit)")
                n196 = call-poly "VISA Configure Serial Port"("VISA resource name"=w348, "Enable Termination\nChar (T)"=FALSE ("Enable Termination\nChar (T)"), "baud rate (9600)"=w347, "data bits (8)"=u16 8, "parity (0:none)"=enum16{"None", "Odd", "Even", "Mark", "Space"}."None", "stop bits (10: 1 bit)"=w351, "flow control (0:none)"=w352) -> ("VISA resource name out"=w346:refnum<visa-resource-name>, "error out"=w345:errorcluster)  [unwired: 7 in]
                n197 = local read "term"() -> (w357:string)
                n198 = Concatenate Strings(w357, "   Commandes Externes (" ("string"), w353, ") ... " ("string")) -> (w356:string)
                n199 = Unbundle By Name(w345) -> ("status"=w359:bool)
                n200 = local write "term"(w356) -> ()
                n201 = Not(x=w359) -> (.not. x?=w358:bool)
              }
              frame 3 {
                w368 = u16 0 items=["None", "XON/XOFF", "RTS/CTS", "XON/XOFF & RTS/CTS", "DTR/DSR", "XON/XOFF & DTR/DSR"] ("flow control (0:none)")
                w367 = u16 10 items=["1.0"=10, "1.5"=15, "2.0"=20] ("stop bits (10: 1 bit)")
                n202 = call-poly "VISA Configure Serial Port"("VISA resource name"=w364, "Enable Termination\nChar (T)"=FALSE ("Enable Termination\nChar (T)"), "baud rate (9600)"=w363, "data bits (8)"=u16 8, "parity (0:none)"=enum16{"None", "Odd", "Even", "Mark", "Space"}."None", "stop bits (10: 1 bit)"=w367, "flow control (0:none)"=w368) -> ("VISA resource name out"=w362:refnum<visa-resource-name>, "error out"=w361:errorcluster)  [unwired: 7 in]
                n203 = local read "term"() -> (w374:string)
                n204 = Concatenate Strings(w374, "   MC-BonOMM (" ("string"), w370, ") ... " ("string")) -> (w373:string)
                n205 = Unbundle By Name(w361) -> ("status"=w375:bool)
                n206 = local write "term"(w373) -> ()
                n207 = Not(x=w375) -> (.not. x?=w369:bool)
              }
              frame 4 {
                n208 = disable-structure shown="Enabled" {
                  disable-tunnel: w385 -> [w390 w394]
                  disable-tunnel: [w389 w398] -> w384
                  disable-tunnel: [w388 w393] -> w383
                  disable-tunnel: [w387 w395] -> w382
                  disable-tunnel: w376 -> [_ w392]
                  frame Disabled {
                    n209 = call "MicroSlide-Initialize.vi"("VISA resource name"=w390) -> ("VRN OUT"=w387:refnum<visa-resource-name>, "Error OUT"=w388:errorcluster)  [unwired: 13 in]
                    n210 = Unbundle By Name(w388) -> ("status"=w386:bool)
                    n211 = Not(x=w386) -> (.not. x?=w389:bool)
                  }
                  frame Enabled {
                    n212 = call-poly "VISA Configure Serial Port"("VISA resource name"=w394, "timeout (10sec)"=u32 1000, "Enable Termination\nChar (T)"=FALSE ("Enable Termination\nChar (T)"), "baud rate (9600)"=w392) -> ("VISA resource name out"=w395:refnum<visa-resource-name>, "error out"=w393:errorcluster)  [unwired: 10 in]
                    n213 = Unbundle By Name(w393) -> ("status"=w397:bool)
                    n214 = Not(x=w397) -> (.not. x?=w398:bool)
                  }
                }
                n215 = local read "term"() -> (w380:string)
                n216 = Concatenate Strings(w380, "   Lame séparatrice (" ("string"), w381, ") ... " ("string")) -> (w379:string)
                n217 = local write "term"(w379) -> ()
              }
            }
            n218 = case shown="True" w276 {
              tunnel: w275 -> [w293 w300]
              tunnel: [refnum<visa-resource-name> "-1" ("VISA resource name out") w300] -> w274
              tunnel: [w291 w298] -> w272
              tunnel: w269 -> [w290 w298]
              frame False {
                w292 = FALSE ("Ports Series")
                n219 = local read "term"() -> (w296:string)
                n220 = VISA Close(VISA resource name=w293, error in (no error)=w290) -> (error out=w291:errorcluster)
                n221 = local write "Ports Series"(w292) -> ()
                n222 = Concatenate Strings(w296, "Erreur!\n" ("string")) -> (w295:string)
                n223 = local write "Go on ?"(w292) -> ()
                n224 = local write "term"(w295) -> ()
              }
              frame True {
                n225 = local read "term"() -> (w302:string)
                n226 = Concatenate Strings(w302, "OK!\n" ("string")) -> (w301:string)
                n227 = local write "term"(w301) -> ()
              }
            }
          }
          "Array of VISA refnum" <- w257
          "Serial" <- w256
          "Array of Baud Rates" <- w255
          n228 = local read "term"() -> (w267:string)
          n229 = Concatenate Strings(w267, "Test des ports séries utilisés :\n" ("string")) -> (w268:string)
          n230 = local write "term"(w268) -> ()
          n231 = call <vilib>:"Close Config Data.vi"("error in (no error)"=w261, "refnum"=w263) -> ("error out"=→"config error out":errorcluster)  [unwired: 8 in, 1 out]
        }
        frame 10 {
          w419 = "communications" ("section")
          n232 = local read "Array of Files"() -> (w429:path[])
          n233 = Index Array(array=w429, index=0) -> (element=w428:path)
          n234 = call <vilib>:"Open Config Data.vi"("configuration file path"=w428) -> ("error out"=w420:errorcluster, "refnum"=w421:T3)  [unwired: 8 in, 1 out]
          n235 = call-poly <vilib>:"Read Key.vi"("section"=w419, "error in (no error)"=w420, "key"="TCS-IP", "refnum"=w421) -> ("error out"=w422:errorcluster, "value"=w416:string, "refnum out"=w423:T3)  [unwired: 4 in, 1 out]
          n236 = call-poly <vilib>:"Read Key.vi"("section"=w419, "error in (no error)"=w422, "key"="TCS-PN", "refnum"=w423) -> ("error out"=w407:errorcluster, "value"=w415:u32, "refnum out"=w408:T3)  [unwired: 4 in, 1 out]
          n237 = To Unsigned Word Integer(number=w415) -> (unsigned 16bit integer=w414:u16)
          n238 = call <vilib>:"Close Config Data.vi"("error in (no error)"=w407, "refnum"=w408) -> ()  [unwired: 8 in, 2 out]
          n239 = local read "term"() -> (w425:string)
          n240 = Concatenate Strings(w425, "Vérification du lien TCP/IP avec TCS ... " ("string")) -> (w426:string)
          n241 = TCP Open Connection(address=w416, remote port or service name=w414, timeout ms (60000)=3000) -> (connection ID=w413:refnum<k5>, error out=w403:errorcluster)  [unwired: 2 in]
          n242 = local write "term"(w426) -> ()
          n243 = Unbundle By Name(w403) -> ("status"=w410:bool)
          n244 = Type Cast(type="", x=w413) -> (*(type *) &x=w411:string)
          n245 = Not(x=w410) -> (.not. x?=w405:bool)
          "TCS" <- w405
          n246 = Type Cast(type=refnum<visa-resource-name> "-1" ("Table VRN"), x=w411) -> (*(type *) &x=w404:refnum<visa-resource-name>)
          n247 = case shown="False" w405 {
            selector: w405 -> [w430 _]
            frame False {
              n248 = local write "Go on ?"(w430) -> ()
            }
            frame True {
            }
          }
          n249 = call-poly "PolyCommError.vi"("VISA IN"=w404, "error IN"=w403) -> ("VISA OUT"=w402:refnum<visa-resource-name>, "error OUT"=w399:errorcluster)  [unwired: 11 in, 1 out]
          "TCS-CommVRN" <- w402
          n250 = local read "Array of VISA refnum"() -> (w401:refnum<visa-resource-name>[])
          n251 = Build Array (concatenate)(w401, w402) -> (w400:refnum<visa-resource-name>[])
          n252 = local write "Array of VISA refnum"(w400) -> ()
          n253 = local write "TCP Error"(w399) -> ()
        }
        frame 11 {
          n254 = local read "TCS"() -> (w431:bool)
          n255 = Select(t="OK!\n" ("string"), s=w431, f="Erreur!\n" ("string")) -> (s? t:f=w434:string)
          n256 = local read "term"() -> (w435:string)
          n257 = Concatenate Strings(w435, w434) -> (w436:string)
          n258 = local write "term"(w436) -> ()
        }
        frame 12 {
          w463 = "communications" ("section")
          n259 = local read "Array of Files"() -> (w470:path[])
          n260 = Index Array(array=w470, index=0) -> (element=w469:path)
          n261 = call <vilib>:"Open Config Data.vi"("configuration file path"=w469) -> ("error out"=w464:errorcluster, "refnum"=w465:T3)  [unwired: 8 in, 1 out]
          n262 = call-poly <vilib>:"Read Key.vi"("section"=w463, "error in (no error)"=w464, "key"="PRAMMS-IP", "refnum"=w465) -> ("error out"=w466:errorcluster, "value"=w454:string, "refnum out"=w467:T3)  [unwired: 4 in, 1 out]
          n263 = local read "Array of Folders"() -> (w441:path[])
          n264 = call-poly <vilib>:"Read Key.vi"("section"=w463, "error in (no error)"=w466, "key"="PRAMMS-PN", "refnum"=w467) -> ("error out"=w456:errorcluster, "value"=w460:u32, "refnum out"=w457:T3)  [unwired: 4 in, 1 out]
          n265 = Index Array(array=w441, index=0) -> (element=w439:path)
          n266 = call <vilib>:"Close Config Data.vi"("error in (no error)"=w456, "refnum"=w457) -> ()  [unwired: 8 in, 2 out]
          n267 = To Unsigned Word Integer(number=w460) -> (unsigned 16bit integer=w453:u16)
          n268 = Build Path(base path=w439, name or relative path="command.ini") -> (appended path=w437:path)
          n269 = call "SAOMM-connect.vi"("IP"=w454, "Port"=w453, "Signature"=u32 1886544237, "Command.ini"=w437) -> ("connection ID"=w452:refnum<k5>, "Connexion"=w451:bool, "Lecture"=w450:bool, "Écriture"=w449:bool, "Error OUT"=w446:errorcluster)  [unwired: 7 in]
          n270 = local read "term"() -> (w472:string)
          n271 = Concatenate Strings(w472, "Vérification du lien avec PRAMMS ... " ("string")) -> (w473:string)
          n272 = local write "term"(w473) -> ()
          n273 = Type Cast(type="", x=w452) -> (*(type *) &x=w458:string)
          n274 = Compound Arithmetic op=AND(w451, w450, w449) -> (w448:bool)
          "PRAMMS" <- w448
          n275 = Type Cast(type=refnum<visa-resource-name> "-1" ("Table VRN"), x=w458) -> (*(type *) &x=w445:refnum<visa-resource-name>)
          n276 = call-poly "PolyCommError.vi"("VISA IN"=w445, "error IN"=w446) -> ("VISA OUT"=w442:refnum<visa-resource-name>)  [unwired: 11 in, 2 out]
          "PRAMMS VRN" <- w442
          n277 = case shown="False" w448 {
            selector: w448 -> [w474 _]
            frame False {
              n278 = local write "Go on ?"(w474) -> ()
            }
            frame True {
            }
          }
          n279 = local read "Array of VISA refnum"() -> (w444:refnum<visa-resource-name>[])
          n280 = Build Array (concatenate)(w444, w442) -> (w443:refnum<visa-resource-name>[])
          n281 = local write "Array of VISA refnum"(w443) -> ()
        }
        frame 13 {
          n282 = local read "PRAMMS"() -> (w475:bool)
          n283 = Select(t="OK!\n" ("string"), s=w475, f="Erreur!\n" ("string")) -> (s? t:f=w478:string)
          n284 = local read "term"() -> (w479:string)
          n285 = Concatenate Strings(w479, w478) -> (w480:string)
          n286 = local write "term"(w480) -> ()
        }
        frame 14 {
          w507 = "communications" ("section")
          n287 = local read "Array of Files"() -> (w514:path[])
          n288 = Index Array(array=w514, index=0) -> (element=w513:path)
          n289 = call <vilib>:"Open Config Data.vi"("configuration file path"=w513) -> ("error out"=w508:errorcluster, "refnum"=w509:T3)  [unwired: 8 in, 1 out]
          n290 = call-poly <vilib>:"Read Key.vi"("section"=w507, "error in (no error)"=w508, "key"="PRAMMS-IP", "refnum"=w509) -> ("error out"=w510:errorcluster, "value"=w498:string, "refnum out"=w511:T3)  [unwired: 4 in, 1 out]
          n291 = local read "Array of Folders"() -> (w485:path[])
          n292 = call-poly <vilib>:"Read Key.vi"("section"=w507, "error in (no error)"=w510, "key"="PRAMMS-PN", "refnum"=w511) -> ("error out"=w500:errorcluster, "value"=w504:u32, "refnum out"=w501:T3)  [unwired: 4 in, 1 out]
          n293 = Index Array(array=w485, index=0) -> (element=w483:path)
          n294 = To Unsigned Word Integer(number=w504) -> (unsigned 16bit integer=w497:u16)
          n295 = Build Path(base path=w483, name or relative path="command.ini") -> (appended path=w481:path)
          n296 = call <vilib>:"Close Config Data.vi"("error in (no error)"=w500, "refnum"=w501) -> ()  [unwired: 8 in, 2 out]
          n297 = local read "term"() -> (w516:string)
          n298 = Concatenate Strings(w516, "Vérification du lien avec l'Hexapode ... " ("string")) -> (w517:string)
          n299 = local write "term"(w517) -> ()
          n300 = call "Hexapod-connect.vi"("IP"=w498, "Port"=w497, "Signature"=u32 1886544237, "path_config"=w481) -> ("connection ID"=w496:refnum<k5>, "Connexion"=w495:bool, "Lecture"=w494:bool, "Écriture"=w493:bool, "Error OUT"=w491:errorcluster)  [unwired: 7 in]
          n301 = Type Cast(type="", x=w496) -> (*(type *) &x=w502:string)
          n302 = Compound Arithmetic op=AND(w495, w494, w493) -> (w489:bool)
          "Hexapode" <- w489
          n303 = Type Cast(type=refnum<visa-resource-name> "-1" ("Table VRN"), x=w502) -> (*(type *) &x=w490:refnum<visa-resource-name>)
          n304 = call-poly "PolyCommError.vi"("VISA IN"=w490, "error IN"=w491) -> ("VISA OUT"=w486:refnum<visa-resource-name>)  [unwired: 11 in, 2 out]
          "Hexapod VRN" <- w486
          n305 = local read "Array of VISA refnum"() -> (w488:refnum<visa-resource-name>[])
          n306 = case shown="False" w489 {
            selector: w489 -> [w518 _]
            frame False {
              n307 = local write "Go on ?"(w518) -> ()
            }
            frame True {
            }
          }
          n308 = Build Array (concatenate)(w488, w486) -> (w487:refnum<visa-resource-name>[])
          n309 = local write "Array of VISA refnum"(w487) -> ()
        }
        frame 15 {
          n310 = local read "Hexapode"() -> (w519:bool)
          n311 = Select(t="OK!\n" ("string"), s=w519, f="Erreur!\n" ("string")) -> (s? t:f=w522:string)
          n312 = local read "term"() -> (w523:string)
          n313 = Concatenate Strings(w523, w522) -> (w524:string)
          n314 = local write "term"(w524) -> ()
        }
        frame 16 {
          n315 = flat-sequence {
            tunnel: [w539] -> w533
            tunnel: [w537] -> w532
            tunnel: [w540] -> w530
            tunnel: [w539] -> w529
            tunnel: [w537] -> w526
            tunnel: w533 -> [w559]
            tunnel: w532 -> [w558]
            tunnel: [w557] -> w531
            tunnel: w530 -> [_]
            tunnel: w529 -> [w556]
            tunnel: [w556] -> w528
            tunnel: [w555] -> w527
            tunnel: w526 -> [w554]
            tunnel: [w554] -> w525
            tunnel: w531 -> [w565]
            tunnel: w528 -> [w566]
            tunnel: w527 -> [w562]
            tunnel: w525 -> [w564]
            frame #0 {
              w545 = "communications" ("section")
              n316 = local read "Array of Files"() -> (w536:path[])
              n317 = Index Array(array=w536, index=0) -> (element=w534:path)
              n318 = call <vilib>:"Open Config Data.vi"("configuration file path"=w534) -> ("error out"=w546:errorcluster, "refnum"=w547:T3)  [unwired: 8 in, 1 out]
              n319 = call-poly <vilib>:"Read Key.vi"("section"=w545, "error in (no error)"=w546, "key"="cRIO-PN" ("section"), "refnum"=w547) -> ("error out"=w548:errorcluster, "value"=w538:u32, "refnum out"=w549:T3)  [unwired: 4 in, 1 out]
              n320 = To Unsigned Word Integer(number=w538) -> (unsigned 16bit integer=w537:u16)
              n321 = local read "term"() -> (w551:string)
              n322 = call-poly <vilib>:"Read Key.vi"("section"=w545, "error in (no error)"=w548, "key"="cRIO-IP" ("section"), "refnum"=w549) -> ("error out"=w541:errorcluster, "value"=w539:string, "refnum out"=w542:T3)  [unwired: 4 in, 1 out]
              n323 = Concatenate Strings(w551, "Connexion à la station météo ... " ("string")) -> (w552:string)
              n324 = local write "term"(w552) -> ()
              n325 = call <vilib>:"Close Config Data.vi"("error in (no error)"=w541, "refnum"=w542) -> ("error out"=w540:errorcluster)  [unwired: 8 in, 1 out]
            }
            frame #1 {
              n326 = TCP Open Connection(address=w559, remote port or service name=w558, timeout ms (60000)=3000) -> (connection ID=w555:refnum<k5>, error out=w561:errorcluster)  [unwired: 2 in]
              n327 = Unbundle By Name(w561) -> ("status"=w560:bool)
              n328 = Not(x=w560) -> (.not. x?=w557:bool)
            }
            frame #2 {
              n329 = case shown="False" w565 {
                tunnel: w562 -> [_ _]
                frame False {
                  n330 = local read "term"() -> (w571:string)
                  n331 = Concatenate Strings(w571, "Erreur!\n" ("string")) -> (w570:string)
                  n332 = local write "Go on ?"(FALSE) -> ()
                  n333 = local write "term"(w570) -> ()
                }
                frame True {
                  n334 = local read "term"() -> (w574:string)
                  n335 = Concatenate Strings(w574, "OK!\n" ("string")) -> (w573:string)
                  n336 = local write "term"(w573) -> ()
                }
              }
              n337 = disable-structure shown="Disabled" {
                disable-tunnel: w562 -> [w568 _]
                frame Disabled {
                  n338 = TCP Close Connection(connection ID=w568) -> (error out=→"TCP Error":errorcluster)  [unwired: 2 in, 1 out]
                }
                frame Enabled {
                }
              }
              n339 = Bundle("value"=w566, w564, "connection ID"=w562, w565) -> (w563:T4)  [unwired: 1 in]
              n340 = local write "Bundle-Meteo"(w563) -> ()
            }
          }
        }
        frame 17 {
          w599 = "chemins"
          n341 = local read "Array of Files"() -> (w584:path[])
          n342 = Index Array(array=w584, index=0) -> (element=w585:path)
          n343 = call <vilib>:"Open Config Data.vi"("configuration file path"=w585) -> ("error out"=w602:errorcluster, "refnum"=w603:T3)  [unwired: 8 in, 1 out]
          n344 = call-poly <vilib>:"Read Key.vi"("section"=w599, "error in (no error)"=w602, "key"="wgetexec", "refnum"=w603) -> ("error out"=w604:errorcluster, "value"=w581:path, "refnum out"=w605:T3)  [unwired: 4 in, 1 out]
          n345 = flat-sequence {
            tunnel: w581 -> [w631]
            tunnel: [w630] -> w594
            tunnel: [w629] -> w576
            tunnel: w596 -> [w634]
            tunnel: [w633] -> w595
            tunnel: [w632] -> w577
            frame #0 {
              n346 = File/Directory Info(path=w631) -> (error out=w630:errorcluster, resolved path=w629:path)  [unwired: 1 in, 5 out]
            }
            frame #1 {
              n347 = File/Directory Info(path=w634) -> (error out=w633:errorcluster, resolved path=w632:path)  [unwired: 1 in, 5 out]
            }
          }
          n348 = call-poly <vilib>:"Read Key.vi"("section"=w599, "error in (no error)"=w604, "key"="idlexec", "refnum"=w605) -> ("error out"=w600:errorcluster, "value"=w596:path, "refnum out"=w601:T3)  [unwired: 4 in, 1 out]
          n349 = local read "term"() -> (w589:string)
          n350 = Concatenate Strings(w589, "Vérification de l'existence des applications externes ... " ("string")) -> (w590:string)
          n351 = call <vilib>:"Close Config Data.vi"("error in (no error)"=w600, "refnum"=w601) -> ("error out"=→"error out":errorcluster, "file path"=w582:path)  [unwired: 8 in]
          n352 = local write "term"(w590) -> ()
          n353 = Unbundle By Name(w594) -> ("status"=w592:bool)
          n354 = Unbundle By Name(w595) -> ("status"=w593:bool)
          n355 = Not(x=w593) -> (.not. x?=w591:bool)
          n356 = Not(x=w592) -> (.not. x?=w583:bool)
          n357 = local write "wget"(w583) -> ()
          n358 = local write "IDL"(w591) -> ()
          n359 = case shown="True" w583 {
            tunnel: w582 -> [_ w615]
            tunnel: w581 -> [_ w617]
            tunnel: [path "" w614] -> w578
            frame False {
            }
            frame True {
              n360 = local read "Array of Folders"() -> (w612:path[])
              n361 = call "Get_properties.vi"("Keyword"="queuelib" ("Section"), "Section"="chemins", "properties.ini"=w615) -> ("string"=w618:string)  [unwired: 6 in, 2 out]
              n362 = Index Array(array=w612, index=2) -> (element=w611:path)
              n363 = Path To String(path=w617) -> (string=w608:string)
              n364 = Concatenate Strings(w608, " --timeout=5 --tries=1" ("string"), " --http-user=carpe", " --http-password=noctem ", w618) -> (w619:string)
              "concatenated string" <- w619
              n365 = call <vilib>:"System Exec.vi"("run minimized? (F)"=TRUE, "working directory"=w611, "command line"=w619) -> ("error out"=w616:errorcluster, "standard error"=→"standard error":string, "standard output"=→"standard output":string)  [unwired: 5 in, 1 out]
              n366 = case shown="Error" w616 {
                tunnel: w611 -> [w627 _]
                tunnel: [w625 path ""] -> w614
                frame No Error {
                  n367 = Build Path(base path=w627, name or relative path="table_technicien.dat") -> (appended path=w625:path)
                }
                frame Error {
                }
              }
            }
          }
          n368 = local read "Array of Files"() -> (w579:path[])
          n369 = Build Array (concatenate)(w579, w578, w577, w576) -> (w580:path[])
          n370 = local write "Array of Files"(w580) -> ()
        }
        frame 18 {
          n371 = local read "wget"() -> (w641:bool)
          n372 = local read "IDL"() -> (w642:bool)
          n373 = And(x=w642, y=w641) -> (x .and. y?=w635:bool)
          n374 = Select(t="OK!\n" ("string"), s=w635, f="Erreur!\n" ("string")) -> (s? t:f=w636:string)
          n375 = case shown="False" w635 {
            selector: w635 -> [w643 _]
            frame False {
              n376 = local write "Go on ?"(w643) -> ()
            }
            frame True {
            }
          }
          n377 = local read "term"() -> (w640:string)
          n378 = Concatenate Strings(w640, w636) -> (w639:string)
          n379 = local write "term"(w639) -> ()
        }
        frame 19 {
          # "VIs requierant une référence ou dont la face avant doit être caché"
          n380 = for {
            tunnel: string[] ["GUI\\CameraTuning.vi", "GUI\\Mode sync(pop-up).vi", "GUI\\InstrChoice.vi"] -> [w670] mode=indexing
            tunnel: [w665] -> w645 mode=indexing
            tunnel: [w664] -> w644 mode=indexing
            i -> [w659]
            n381 = local read "Array of Folders"() -> (w663:path[])
            n382 = Index Array(array=w663, index=4) -> (element=w662:path)
            n383 = Build Path(base path=w662, name or relative path=w670) -> (appended path=w669:path)
            n384 = Open VI Reference(vi path=w669) -> (vi reference=w660:refnum<vi>, error out=w658:errorcluster)  [unwired: 5 in]
            n385 = case shown="0" w659 {
              tunnel: w660 -> [_ w672 _ _]
              tunnel: w658 -> [_ w671 _ _]
              frame -1, Default {
              }
              frame 0 {
                n386 = case shown="No Error" w671 {
                  tunnel: w672 -> [w673 _]
                  frame No Error {
                    n387 = global write "Globals.vi" "CameraTuning VI Refnum"(w673) -> ()
                  }
                  frame Error {
                  }
                }
              }
              frame 1 {
              }
              frame 2 {
              }
            }
            n388 = property class="VI"(reference=w660, error in=w658) -> (reference out=w667:refnum<vi>, error out=w666:errorcluster, "Front Panel.Open"=w668:bool)
            n389 = case shown="True" w668 {
              tunnel: w667 -> [w675 w680]
              tunnel: [w675 w679] -> w665
              tunnel: w666 -> [w674 w677]
              tunnel: [w674 w676] -> w664
              frame False {
              }
              frame True {
                n390 = property class="VI"(reference=w680, error in=w677, "Front Panel.Open"=FALSE) -> (reference out=w679:refnum<vi>, error out=w676:errorcluster)
              }
            }
          }
          n391 = local read "term"() -> (w647:string)
          n392 = Concatenate Strings(w647, "Vérification de l'état des sous-vis ... " ("string")) -> (w648:string)
          n393 = local write "term"(w648) -> ()
          n394 = flat-sequence {
            tunnel: w645 -> [_]
            tunnel: w644 -> [w653]
            frame #0 {
              n395 = for {
                tunnel: w653 -> [w657] mode=indexing
                tunnel: [w656] -> w652 mode=indexing
                n396 = Unbundle By Name(w657) -> ("status"=w656:bool)
              }
              n397 = disable-structure shown="Disabled" {
                frame Disabled {
                  n398 = Wait (ms)(milliseconds to wait=u32 500) -> ()  [unwired: 1 out]
                }
                frame Enabled {
                }
              }
              n399 = Boolean Array To Number(Boolean array=w652) -> (number=w651:u32)
              n400 = Greater Than 0?(x=w651) -> (x > 0?=w650:bool)
              n401 = case shown="True" w650 {
                frame False {
                }
                frame True {
                  w655 = FALSE
                  n402 = local write "Go on ?"(w655) -> ()
                  n403 = local write "SubVIs"(w655) -> ()
                }
              }
            }
          }
        }
        frame 20 {
          n404 = local read "SubVIs"() -> (w681:bool)
          n405 = Select(t="OK!\n" ("string"), s=w681, f="Erreur!\n" ("string")) -> (s? t:f=w684:string)
          n406 = local read "term"() -> (w685:string)
          n407 = Concatenate Strings(w685, w684) -> (w686:string)
          n408 = local write "term"(w686) -> ()
        }
        frame 21 {
          # "Mettre à la fin pour recommencer tout ..."
          n409 = local read "Go on ?"() -> (w689:bool)
          n410 = case shown="True" w689 {
            tunnel: [w709 FALSE ("true")] -> w690
            frame False {
              w708 = T2."Enabled" ("Disabled")
              n411 = disable-structure shown="Enabled" {
                disable-tunnel: [w710 TRUE ("true")] -> w709
                frame Disabled {
                  n412 = One Button Dialog(message="Une ou plusieurs erreurs se sont produites lors de l'initialisation.\nVous pouvez annuler l'ouverture du programme, recommencez l'initialisation ou ignorer les erreurs.\n\nCependant, si vous ignorez les erreurs, il se peut que \ncertaines fonctionnalités ne soient pas disponibles") -> (true=w710:bool)  [unwired: 1 in]
                }
                frame Enabled {
                }
              }
              n413 = property on="cancel" class="Bool (strict)"("DisabledEnum"=w708) -> ()  [unwired: 2 in, 2 out]
              n414 = property on="ignore" class="Bool"("DisabledEnum"=w708) -> ()  [unwired: 2 in, 2 out]
              n415 = property on="restart" class="Bool"("DisabledEnum"=w708) -> ()  [unwired: 2 in, 2 out]
            }
            frame True {
            }
          }
          n416 = local read "term"() -> (w688:string)
          n417 = case shown="False" w690 {
            tunnel: w688 -> [_ w692]
            tunnel: [_ w691] -> w687
            frame False {
            }
            frame True {
              n418 = while {
                tunnel: w692 -> [w703]
                tunnel: ["restart"] -> w691
                i -> [w706]
                stop <- w695 stop-if-true
                n419 = Quotient & Remainder(x=w706, y=10) -> (x-y*floor(x/y)=w699:i32)  [unwired: 1 out]
                n420 = Wait (ms)(milliseconds to wait=u32 100) -> ()  [unwired: 1 out]
                n421 = Less?(x=w699, y=6) -> (x < y?=w698:bool)
                n422 = Select(t="\nEn attente de la réponse de l'usagé ..." ("string"), s=w698, f="") -> (s? t:f=w701:string)
                n423 = local read "cancel"() -> (w696:bool)
                n424 = Concatenate Strings(w703, w701) -> (w702:string)
                n425 = Compound Arithmetic op=OR(w696, "restart", "ignore") -> (w695:bool)
                n426 = local write "Go on ?"("ignore") -> ()
                n427 = local write "term"(w702) -> ()
              }
            }
          }
        }
        frame 22.. {
          n428 = local read "Go on ?"() -> (w715:bool)
          n429 = case shown="True" w715 {
            tunnel: [_ TRUE] -> w714
            frame False {
            }
            frame True {
              n430 = local read "term"() -> (w717:string)
              n431 = Concatenate Strings(w717, "\nVérifications complétées\nBonne Nuit !!!" ("string")) -> (w720:string)
              n432 = local write "term"(w720) -> ()
              n433 = disable-structure shown="Enabled" {
                frame Disabled {
                  n434 = Wait (ms)(milliseconds to wait=u32 666) -> ()  [unwired: 1 out]
                }
                frame Enabled {
                  n435 = Wait (ms)(milliseconds to wait=u32 200) -> ()  [unwired: 1 out]
                }
                frame Disabled {
                }
              }
              "SkipInstr" <- "SkipInstr"
            }
          }
        }
      }
      n436 = Or(x="cancel", y=w10) -> (x .or. y?=w12:bool)
    }
  }
  n437 = disable-structure shown="Disabled" {
    frame Disabled {
      n438 = flat-sequence {
        tunnel: w740 -> [w743]
        tunnel: [w743] -> w723
        frame #0 {
          n439 = Wait (ms)(milliseconds to wait=u32 500) -> ()  [unwired: 1 out]
        }
      }
      n440 = call "MC-BonOMM_talker.vi"("MC-BonOMM VRN"=w723, "Commande"="m", "byte count"=u32 1, "Timeout (ms)"=3000, "answer=command?"=FALSE) -> ("Answer"=w725:string, "ok ?"=w726:bool)
      n441 = VISA Write(write buffer="r" ("Commande")) -> (VISA resource name out=w738:refnum<visa-resource-name>)  [unwired: 2 in, 2 out]
      n442 = property class="Instr"(reference=w738) -> (reference out=w737:refnum<visa-resource-name>, "Serial Settings:Number of Bytes at Serial Port"=w736:u32)  [unwired: 1 in, 1 out]
      n443 = Equal?(x="f", y=w725) -> (x = y?=w730:bool)
      n444 = Equal?(x=w725, y="x") -> (x = y?=w731:bool)
      n445 = Or(x=w730, y=w731) -> (x .or. y?=w727:bool)
      n446 = And(x=w727, y=w726) -> (x .and. y?=w724:bool)
      n447 = VISA Read(VISA resource name=w737, byte count=w736) -> (VISA resource name out=w740:refnum<visa-resource-name>)  [unwired: 1 in, 3 out]
      n448 = case shown="True" w724 {
        tunnel: [w744 w758] -> w741
        tunnel: w740 -> [_ w749]
        frame False {
          n449 = Two Button Dialog(message="MC-BonOMM n'a pas été détecté !\nSouhaitez-vous recommencer l'initalisation ?", 1:"NON" ("F button name (\"Cancel\")"), 2:"OUI" ("T button name (\"OK\")")) -> (T button?=w745:bool)
          n450 = Not(x=w745) -> (.not. x?=w744:bool)
        }
        frame True {
          n451 = call <vilib>:"Three Button Dialog.vi"("Allow user to close window? (TRUE)"=FALSE, "Justify Message (Left)"=enum16{"Left", "Center", "Right"}."Center", "Right Button Text (\"Cancel\")"="Foyer ST-133" ("F button name (\"Cancel\")"), "Center Button Text (\"No\")"="RàF (PANO-II)" ("F button name (\"Cancel\")"), "Left Button Text (\"Yes\")"="RàF (BonOMM)" ("T button name (\"OK\")"), "message"="MC-BonOMM a été détecté !\nQuel mode souhaité vous utiliser ?") -> ("Which Button?"=w751:T5)  [unwired: 5 in]
          n452 = case shown="\"Left Button\", Default" w751 {
            tunnel: ["o" "x" "f"] -> w750
            frame "Center Button" {
            }
            frame "Right Button" {
            }
            frame "Left Button", Default {
            }
          }
          n453 = call "MC-BonOMM_talker.vi"("MC-BonOMM VRN"=w749, "Commande"=w750, "Timeout (ms)"=1000, "answer=command?"=TRUE) -> ("ok ?"=w758:bool)  [unwired: 1 in, 1 out]
        }
      }
    }
    frame Enabled {
    }
  }
